vi "GC Vacuum - Step 7.vi"(7 "Step":i32, 8 "error in":errorcluster, 9 "Test Results In":T8, 10 "Gas":T1, 11 "GC Configuration":T2) -> (0 "error out":errorcluster, 1 "Test Results Out":T8, 2 "Gas Out":T1 caption="Gas", 3 "GC Configuration Out":T2)   [LabVIEW 2015]
uses:
  Controls/Test Information.ctl
  Controls/Vacuum Test.ctl
  Controls/Test Timing.ctl
  Controls/Vaccum Thresholds.ctl
  Controls/Helium Test.ctl
  Controls/Helium Thresholds.ctl
  CAN Communication/Gas/Typedefs/Session Handle.ctl
  CAN Communication/Gas/Gas.lvclass
  Controls/Test Results.ctl
  Controls/Step Result.ctl
  CAN Communication/Gas/Typedefs/Valves.ctl
  SubVIs/Timing/Timing.lvlib
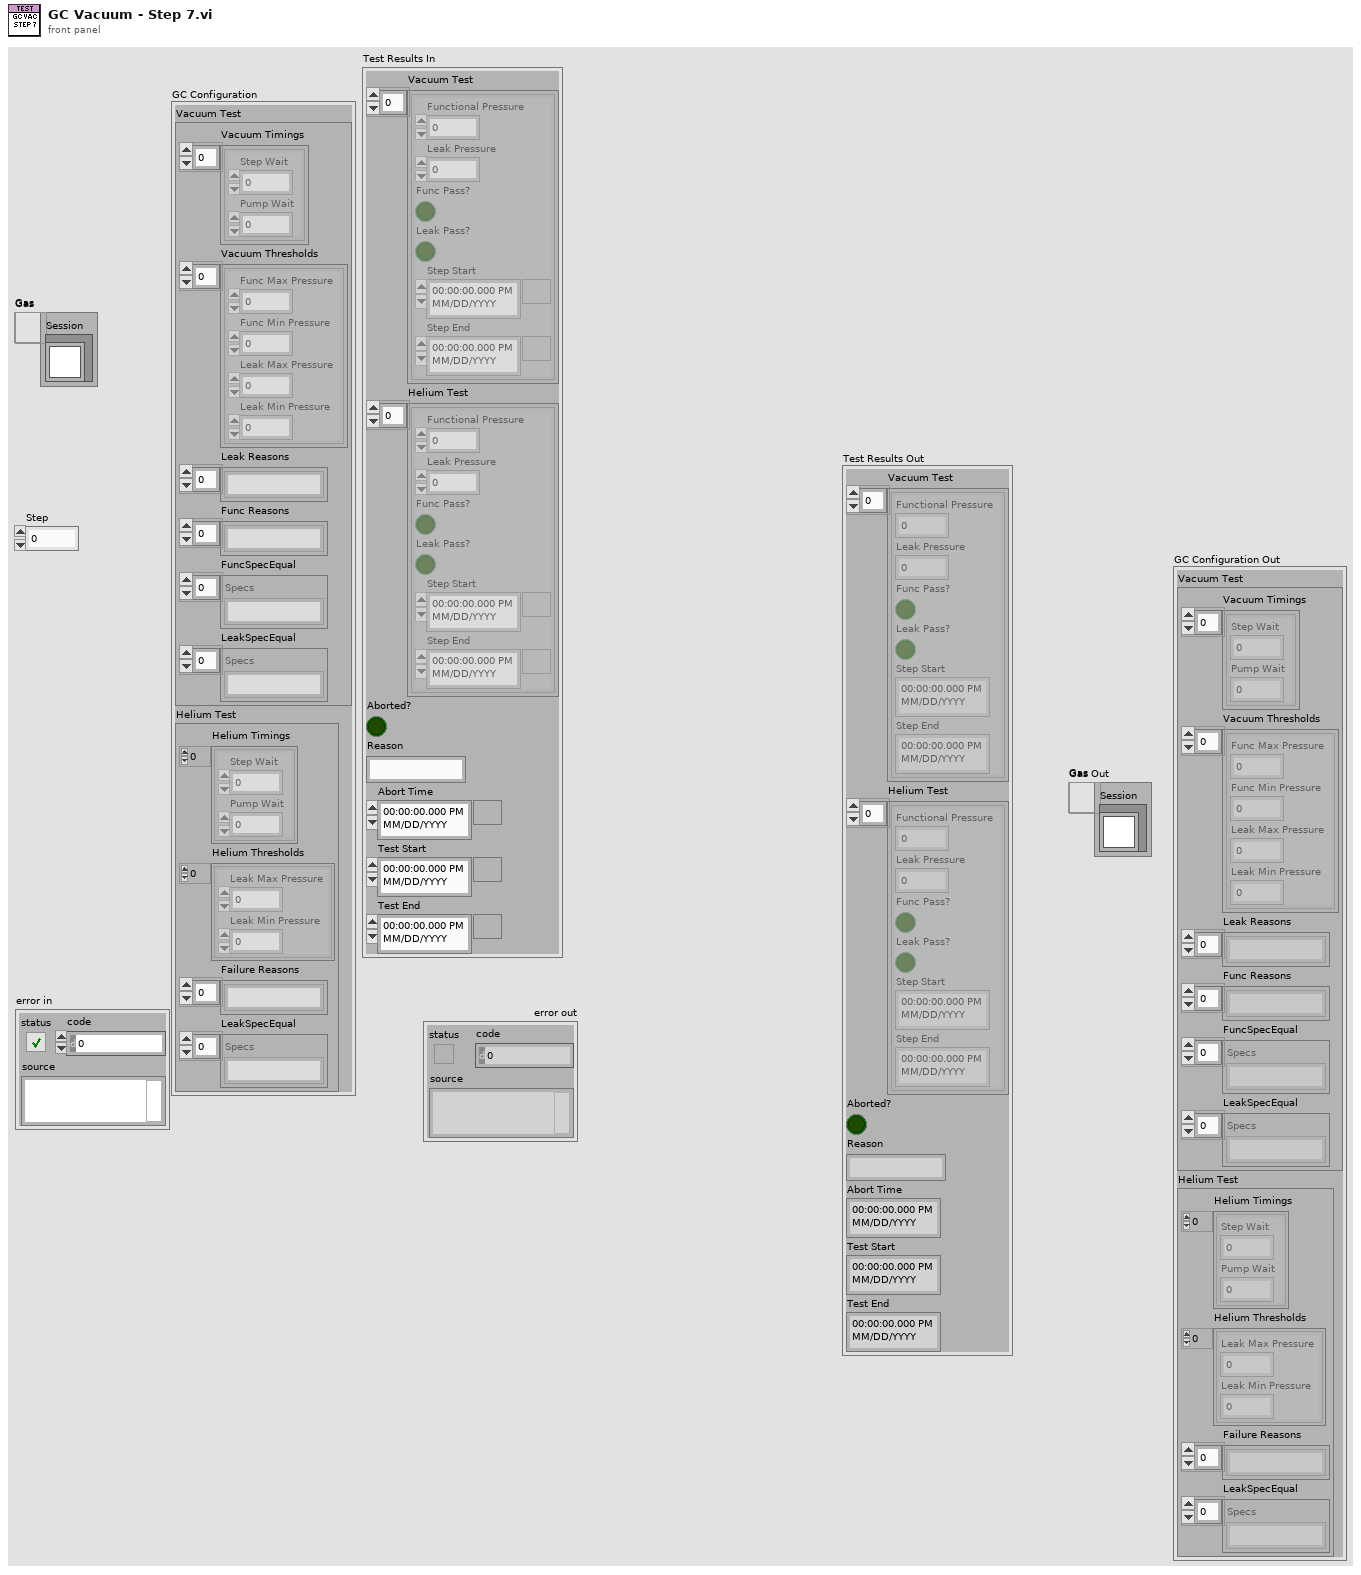
[diagram p1: front panel]
types:
  T1 = typedef "Gas.lvclass/Session Handle.ctl" = refnum<data-value>
  T2 = typedef "Test Information.ctl" = cluster{"Vacuum Test":T3, "Helium Test":T6}
  T3 = typedef "Vacuum Test.ctl" = cluster{"Vacuum Timings":T4[], "Vacuum Thresholds":T5[], "Leak Reasons":string[], "Func Reasons":string[], "FuncSpecEqual":string[], "LeakSpecEqual":string[]}
  T4 = typedef "Test Timing.ctl" = cluster{"Step Wait":dbl, "Pump Wait":dbl}
  T5 = typedef "Vaccum Thresholds.ctl" = cluster{"Func Max Pressure":dbl, "Func Min Pressure":dbl, "Leak Max Pressure":dbl, "Leak Min Pressure":dbl}
  T6 = typedef "Helium Test.ctl" = cluster{"Helium Timings":T4[], "Helium Thresholds":T7[], "Failure Reasons":string[], "LeakSpecEqual":string[]}
  T7 = typedef "Helium Thresholds.ctl" = cluster{"Leak Max Pressure":dbl, "Leak Min Pressure":dbl}
  T8 = typedef "Test Results.ctl" = cluster{"Vacuum Test":T9[], "Helium Test":T9[], "Aborted?":bool, "Reason":string, "Abort Time":timestamp, "Test Start":timestamp, "Test End":timestamp}
  T9 = typedef "Step Result.ctl" = cluster{"Functional Pressure":dbl, "Leak Pressure":dbl, "Func Pass?":bool, "Leak Pass?":bool, "Step Start":timestamp, "Step End":timestamp}
  T10 = typedef "Gas.lvclass/Valves.ctl" = u16
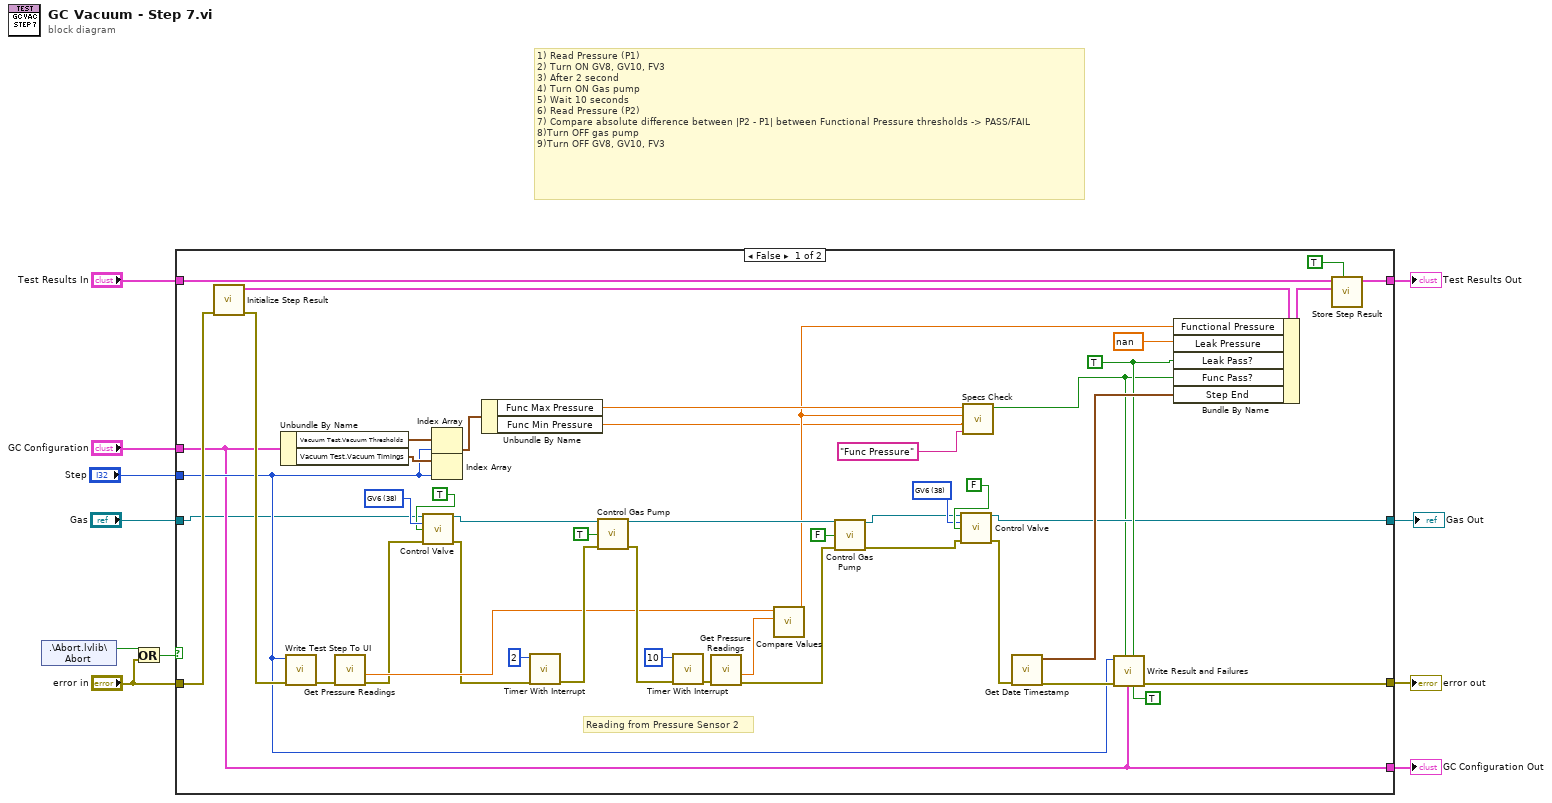
[diagram p0: block diagram]
diagram:
  # "1) Read Pressure (P1)\n2) Turn ON GV8, GV10, FV3\n3) After 2 second\n4) Turn ON Gas pump\n5) Wait 10 seconds\n6) Read Pressure (P2)\n7) Compare absolute difference between |P2 - P1| between Functional Pressure thresholds -> PASS/FAIL\n8)Turn OFF gas pump\n9)Turn OFF GV8, GV10, FV3"
  n1 = shared-variable ".\\Abort.lvlib\\Abort"() -> (w10:bool)  [unwired: 1 in, 1 out]
  n2 = Or(x=w10, y="error in") -> (x .or. y?=w9:bool)
  n3 = case shown="False" w9 {
    tunnel: "error in" -> [w58 w61]
    tunnel: "Test Results In" -> [w55 w62]
    tunnel: [w56 w62] -> w7
    tunnel: [w47 w61] -> w6
    tunnel: "GC Configuration" -> [w45 w60]
    tunnel: "Step" -> [w46 _]
    tunnel: [w45 w60] -> w3
    tunnel: [w19 w59] -> w1
    tunnel: "Gas" -> [w17 w59]
    frame False {
      w23 = T10 38 items=["GV1"=33, "GV2"=34, "GV3"=35, "GV4"=36, "GV5"=37, "GV6"=38, "GV7"=39, "GV8"=40, "GV9"=41, "GV10"=42, "GV11"=43, "LV3"=51, "LV4"=52] ("Valves")
      w26 = T10 38 items=["GV1"=33, "GV2"=34, "GV3"=35, "GV4"=36, "GV5"=37, "GV6"=38, "GV7"=39, "GV8"=40, "GV9"=41, "GV10"=42, "GV11"=43, "LV3"=51, "LV4"=52] ("Valves")
      w34 = TRUE ("In Range?")
      # "Reading from Pressure Sensor 2"
      n4 = call "Initialize Step Result.vi"("error in (no error)"=w58) -> ("error out"=w57:errorcluster, "New Step Result"=w54:T9)  [unwired: 8 in, 1 out]
      n5 = Unbundle By Name(w45) -> ("Vacuum Test.Vacuum Thresholds"=w51:T5[], "Vacuum Test.Vacuum Timings"=w50:T4[])
      n6 = call "Write Test Step To UI.vi"("error in (no error)"=w57, "Step"=w46) -> ("error out"=w44:errorcluster)  [unwired: 9 in]
      n7 = call "Get Pressure Readings.vi"("error in (no error)"=w44) -> ("error out"=w28:errorcluster, "GAS Pressure 2"=w32:dbl)  [unwired: 6 in, 3 out]
      n8 = call "Control Valve.vi"("Session Handle in"=w17, "Valves"=w26, "Energize?"=TRUE, "error in (no error)"=w28) -> ("Session Handle out"=w20:T1, "error out"=w27:errorcluster)  [unwired: 9 in, 1 out]
      n9 = Index Array(array=w51, index=w46) -> (element=w49:T5)
      n10 = Index Array(array=w50, index=w46) -> ()  [unwired: 1 out]
      n11 = Unbundle By Name(w49) -> ("Func Max Pressure"=w15:dbl, "Func Min Pressure"=w13:dbl)
      n12 = call "Timer With Interrupt.vi"("error in (no error)"=w27, "Wait (s)"=2) -> ("error out"=w42:errorcluster)  [unwired: 7 in, 2 out]
      n13 = call "Control Gas Pump.vi"("Session Handle in"=w20, "On?"=TRUE, "error in (no error)"=w42) -> ("Session Handle out"=w36:T1, "error out"=w40:errorcluster)  [unwired: 10 in, 1 out]
      n14 = call "Timer With Interrupt.vi"("error in (no error)"=w40, "Wait (s)"=10) -> ("error out"=w38:errorcluster)  [unwired: 7 in, 2 out]
      n15 = call "Get Pressure Readings.vi"("error in (no error)"=w38) -> ("error out"=w37:errorcluster, "GAS Pressure 2"=w31:dbl)  [unwired: 6 in, 3 out]
      n16 = call "Compare Values.vi"("P2"=w31, "P1"=w32) -> ("Abs Diff"=w14:dbl)  [unwired: 9 in]
      n17 = call "Control Gas Pump.vi"("Session Handle in"=w36, "On?"=FALSE, "error in (no error)"=w37) -> ("Session Handle out"=w18:T1, "error out"=w22:errorcluster)  [unwired: 10 in, 1 out]
      n18 = call "Control Valve.vi"("Session Handle in"=w18, "Valves"=w23, "Energize?"=FALSE, "error in (no error)"=w22) -> ("Session Handle out"=w19:T1, "error out"=w21:errorcluster)  [unwired: 9 in, 1 out]
      n19 = call "Specs Check.vi"("parameter"="Func Pressure", "lower limit"=w13, "x"=w14, "upper limit"=w15) -> ("In Range?"=w16:bool)  [unwired: 6 in, 1 out]
      n20 = call "Get Date Timestamp.vi"("error in (no error)"=w21) -> ("error out"=w48:errorcluster, "current time"=w52:timestamp)  [unwired: 9 in]
      n21 = call "Write Result and Failures.vi"("Vacuum?"=TRUE, "Leak"=w34, "GC Configuration"=w45, "Func"=w16, "error in (no error)"=w48, "Step"=w46) -> ("error out"=w47:errorcluster)  [unwired: 5 in]
      n22 = Bundle By Name(cluster=w54, "Functional Pressure"=w14, "Leak Pressure"=nan ("Step Pressure"), "Leak Pass?"=w34, "Func Pass?"=w16, "Step End"=w52) -> (w53:T9)
      n23 = call "Store Step Result.vi"("Vacuum?"=TRUE, "Step Result"=w53, "Test Results In"=w55) -> ("Test Results Out"=w56:T8)  [unwired: 8 in]
    }
    frame True {
    }
  }
  "error out" <- w6
  "Test Results Out" <- w7
  "GC Configuration Out" <- w3
  "Gas Out" <- w1
